vi "niRFUtil MEAS Waveform Value (complex wfm).vi"(2 "x":sgl format="%^.6e", 3 "Waveform In":T1 {"y" format="%.2f"; "dx" format="%^.2e"; "x0" format="%^.2e"}) -> (1 "Value":csg format="%.2f")   [LabVIEW 2015, in "niRFUtil.lvlib"]
doc: "(c) Copyright 2006, National Instruments, Inc. This VI may not be duplicated, sold, or distributed without written consent from National Instruments."
uses:
  niRFUtil.lvlib
  Includes/niRFUtil INC Complex Waveform.ctl
  Includes/niRFUtil INC Complex Array.ctl
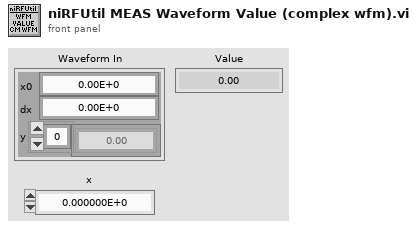
[diagram p1: front panel]
types:
  T1 = typedef "niRFUtil.lvlib/niRFUtil INC Complex Waveform.ctl" = cluster{"x0":dbl, "dx":dbl, "y":T2}
  T2 = typedef "niRFUtil.lvlib/niRFUtil INC Complex Array.ctl" = csg[]
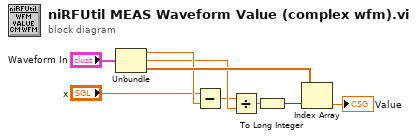
[diagram p0: block diagram]
diagram:
  n1 = Unbundle("Waveform In") -> ("x0"=w8:dbl, "dx"=w7:dbl, "y"=w9:T2)
  n2 = Subtract(x="x", y=w8) -> (x-y=w6:dbl)
  n3 = Divide(x=w6, y=w7) -> (x/y=w5:dbl)
  n4 = To Long Integer(number=w5) -> (32bit integer=w4:i32)
  n5 = Index Array(array=w9, index=w4) -> (element=→"Value":csg)
